vi "array down.vi"(8 "error in (no error)":errorcluster, 11 "Array in":refnum<vi>) -> (0 "error out":errorcluster, 3 "Array out":refnum<vi>)   [LabVIEW 2014, in "Tagbus PID Module editor node.lvclass"]
uses:
  Tagbus PID Module editor node.lvclass
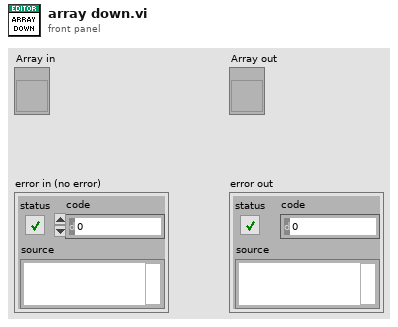
[diagram p1: front panel]
types:
  T1 = cluster{"Loop ID":string, "Tags":cluster{"Setpoint":string, "Process Variable":string, "Output":string}, "Gains":cluster{"P":dbl, "I":dbl, "D":dbl}, "Range":cluster{"High":dbl, "Low":dbl}}[]
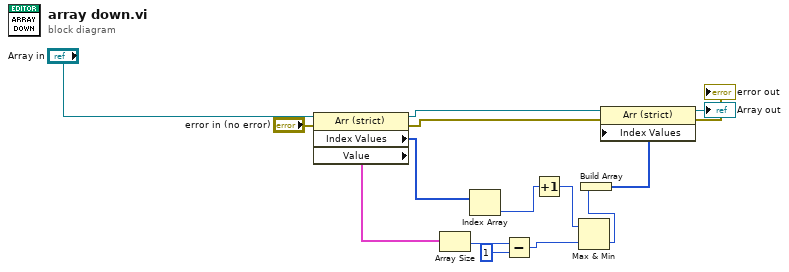
[diagram p0: block diagram]
diagram:
  n1 = property class="Arr (strict)"(reference="Array in", error in="error in (no error)") -> (reference out=w5:refnum<vi>, error out=w12:errorcluster, "Index Values"=w7:u32[], "Value"=w11:T1)
  n2 = Array Size(array=w11) -> (size(s)=w3:i32)
  n3 = Index Array(array=w7) -> (element=w8:u32)  [unwired: 1 in]
  n4 = Subtract(x=w3, y=1) -> (x-y=w1:i32)
  n5 = Increment(x=w8) -> (x+1=w9:u32)
  n6 = Max & Min(x=w9, y=w1) -> (min(x,y)=w10:u32)  [unwired: 1 out]
  n7 = Build Array(w10) -> (w6:u32[])
  n8 = property class="Arr (strict)"(reference=w5, error in=w12, "Index Values"=w6) -> (reference out=→"Array out":refnum<vi>, error out=→"error out":errorcluster)
